vi "Generate VS Channels Info.vi"(10 "Label Format (Decimal)":enum16{"Decimal", "Octal"}(ring), 11 "Transfer Type":enum16{"Acyclic", "Scheduled"}(ring)) -> (0 "Tx Trigger Channels Array":string[](array[string]), 1 "Tx Disable Channels Array":string[](array[string]), 2 "Tx Channels Array":string[](array[string]), 3 "Rx Channels Array":string[](array[string]), 4 "Is First Parameter? Array":bool[](array[boolean]))   [LabVIEW 2020]
uses:
  b281cc4c-f5bf-4263-a2a4-b8c933cd51f6.vi
  9ae52f1a-1e4b-4aa8-8e73-03c214062afe.vi
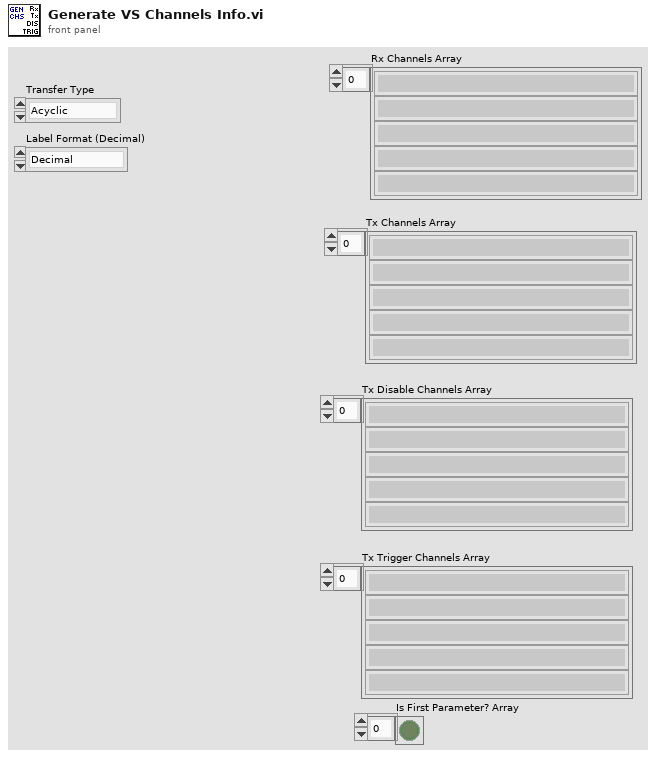
[diagram p1: front panel]
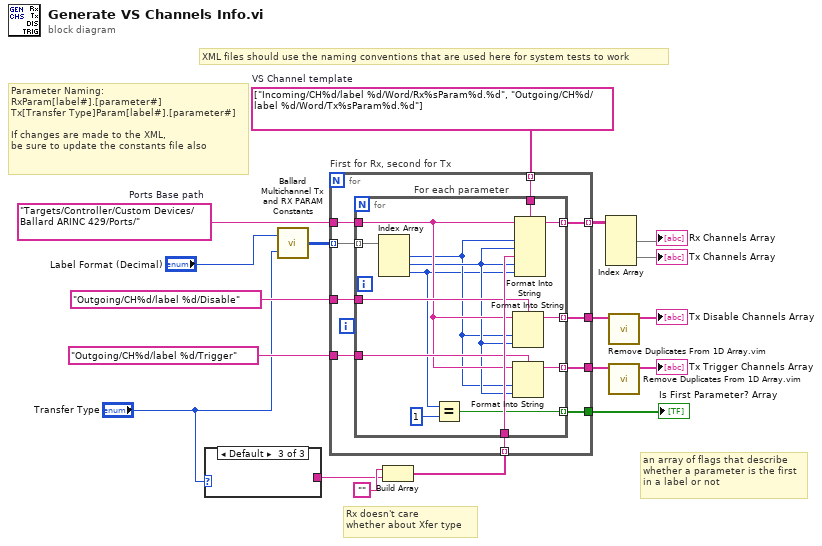
[diagram p0: block diagram]
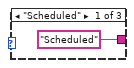
[diagram p2: hidden frame]
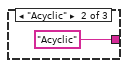
[diagram p3: hidden frame]
diagram:
  w11 = "Targets/Controller/Custom Devices/Ballard ARINC 429/Ports/"  # Ports Base path
  w18 = string[] ["Incoming/CH%d/label %d/Word/Rx%sParam%d.%d", "Outgoing/CH%d/label %d/Word/Tx%sParam%d.%d"]  # VS Channel template
  # "Rx doesn't care\nwhether about Xfer type"
  # "an array of flags that describe\nwhether a parameter is the first\nin a label or not"
  # "Parameter Naming:\nRxParam[label#].[parameter#]\nTx[Transfer Type]Param[label#].[parameter#]\n\nIf changes are made to the XML,\nbe sure to update the constants file also"
  # "XML files should use the naming conventions that are used here for system tests to work"
  n1 = case shown="Default" "Transfer Type" {
    tunnel: ["Scheduled" "Acyclic" _] -> w2
    frame "Scheduled" {
    }
    frame "Acyclic" {
    }
    frame Default {
    }
  }
  n2 = call "Ballard Multichannel Tx and RX PARAM Constants.vi"("Transfer Type"="Transfer Type", "Label Format (Decimal)"="Label Format (Decimal)") -> ("Parameters (3D Array)"=w10:i32[][][])
  n3 = Build Array("", w2) -> (w5:string[])
  n4 = for "First for Rx, second for Tx" {
    tunnel: [w30] -> w4 mode=indexing
    tunnel: w10 -> [w29] mode=indexing
    tunnel: w11 -> [w28]
    tunnel: w18 -> [w27] mode=indexing
    tunnel: w5 -> [w26] mode=indexing
    tunnel: "Outgoing/CH%d/label %d/Disable" ("String") -> [w25]
    tunnel: [w24] -> w13
    tunnel: "Outgoing/CH%d/label %d/Trigger" ("String") -> [w23]
    tunnel: [w22] -> w15
    tunnel: [w21] -> w9
    n5 = for "For each parameter" {
      tunnel: w29 -> [w44] mode=indexing
      tunnel: w27 -> [w43]
      tunnel: [w42] -> w30 mode=indexing
      tunnel: w28 -> [w37]
      tunnel: w26 -> [w41]
      tunnel: w25 -> [w40]
      tunnel: [w39] -> w24 mode=indexing
      tunnel: w23 -> [w38]
      tunnel: [w35] -> w22 mode=indexing
      tunnel: [w31] -> w21 mode=indexing
      n6 = Index Array(array=w44) -> (element #1=w34:i32, element #2=w36:i32, element #3=w32:i32)  [unwired: 3 in]
      n7 = Equal?(x=w32, y=1) -> (x = y?=w31:bool)
      n8 = Format Into String(format string=w40, initial string=w37, w34, w36) -> (resulting string=w39:string)  [unwired: 1 in, 1 out]
      n9 = Format Into String(format string=w38, initial string=w37, w34, w36) -> (resulting string=w35:string)  [unwired: 1 in, 1 out]
      n10 = Format Into String(format string=w43, initial string=w37, w34, w36, w41, w36, w32) -> (resulting string=w42:string)  [unwired: 1 in, 1 out]
    }
  }
  "Is First Parameter? Array" <- w9
  n11 = Index Array(array=w4) -> (element #1=→"Rx Channels Array":string[], element #2=→"Tx Channels Array":string[])  [unwired: 4 in]
  n12 = call "Remove Duplicates From 1D Array.vim"("array"=w13) -> ("array with duplicates removed"=→"Tx Disable Channels Array":string[])  [unwired: 10 in]
  n13 = call "Remove Duplicates From 1D Array.vim"("array"=w15) -> ("array with duplicates removed"=→"Tx Trigger Channels Array":string[])  [unwired: 10 in]
